vi "run control loops.vi"(6 "Reference Temperature [°F]":dbl, 8 "error in":errorcluster, 9 "Frequncy [Hz]":u16, 10 "input cluster":T1, 11 "dt [s]":dbl) -> (0 "error out":errorcluster, 1 "output cluster":T1, 2 "Duty Cycle Array":dbl[](array[numeric]), 3 "Temperature Array":dbl[](array[numeric]))   [LabVIEW 2025]
uses:
  Classes/controller/controller.lvclass
  Classes/hardware/hardware.lvclass
  Classes/data log/data log.lvclass
panel:
  in  "Hardware":refnum<class "hardware.lvclass">
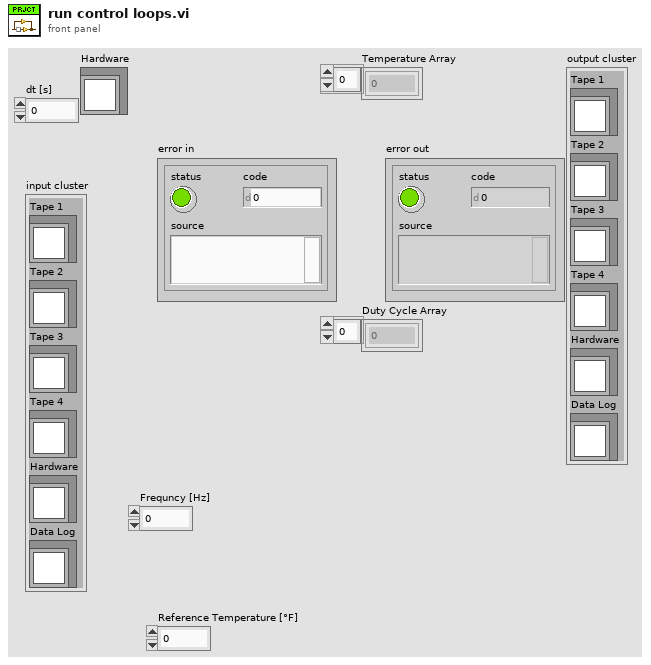
[diagram p1: front panel]
types:
  T1 = cluster{"Tape 1":refnum<class "controller.lvclass">, "Tape 2":refnum<class "controller.lvclass">, "Tape 3":refnum<class "controller.lvclass">, "Tape 4":refnum<class "controller.lvclass">, "Hardware":refnum<class "hardware.lvclass">, "Data Log":refnum<class "data log.lvclass">}
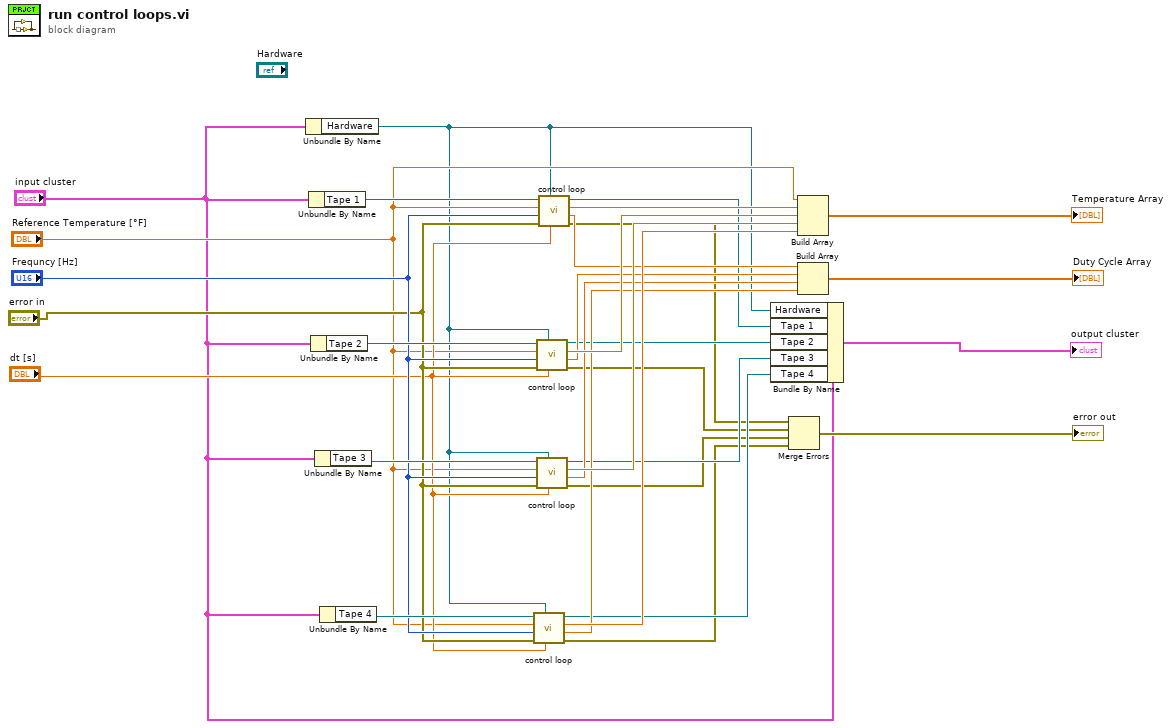
[diagram p0: block diagram]
diagram:
  n1 = Unbundle By Name("input cluster") -> ("Hardware"=w1:refnum<class "hardware.lvclass">)
  n2 = Unbundle By Name("input cluster") -> ("Tape 1"=w30:refnum<class "controller.lvclass">)
  n3 = Unbundle By Name("input cluster") -> ("Tape 2"=w29:refnum<class "controller.lvclass">)
  n4 = Unbundle By Name("input cluster") -> ("Tape 3"=w28:refnum<class "controller.lvclass">)
  n5 = Unbundle By Name("input cluster") -> ("Tape 4"=w27:refnum<class "controller.lvclass">)
  n6 = call-dynamic "control loop.vi"("dt [s]"="dt [s]", "Hardware"=w1, "error in (no error)"="error in", "Frequncey [Hz]"="Frequncy [Hz]", "Reference"="Reference Temperature [°F]", "controller in"=w27) -> ("error out"=w4:errorcluster, "input"=w14:dbl, "State"=w19:dbl, "controller out"=w9:refnum<class "controller.lvclass">)  [unwired: 2 in]
  n7 = call-dynamic "control loop.vi"("dt [s]"="dt [s]", "Hardware"=w1, "error in (no error)"="error in", "Frequncey [Hz]"="Frequncy [Hz]", "Reference"="Reference Temperature [°F]", "controller in"=w29) -> ("error out"=w6:errorcluster, "input"=w16:dbl, "State"=w21:dbl, "controller out"=w11:refnum<class "controller.lvclass">)  [unwired: 2 in]
  n8 = call-dynamic "control loop.vi"("dt [s]"="dt [s]", "Hardware"=w1, "error in (no error)"="error in", "Frequncey [Hz]"="Frequncy [Hz]", "Reference"="Reference Temperature [°F]", "controller in"=w28) -> ("error out"=w5:errorcluster, "input"=w15:dbl, "State"=w20:dbl, "controller out"=w10:refnum<class "controller.lvclass">)  [unwired: 2 in]
  n9 = call-dynamic "control loop.vi"("dt [s]"="dt [s]", "Hardware"=w1, "error in (no error)"="error in", "Frequncey [Hz]"="Frequncy [Hz]", "Reference"="Reference Temperature [°F]", "controller in"=w30) -> ("error out"=w7:errorcluster, "input"=w17:dbl, "State"=w22:dbl, "controller out"=w12:refnum<class "controller.lvclass">)  [unwired: 2 in]
  n10 = Bundle By Name(cluster="input cluster", "Hardware"=w1, "Tape 1"=w12, "Tape 2"=w11, "Tape 3"=w10, "Tape 4"=w9) -> (→"output cluster":T1)
  n11 = Merge Errors(w7, w6, w5, w4) -> (→"error out":errorcluster)
  n12 = Build Array("Reference Temperature [°F]", w22, w21, w20, w19) -> (→"Temperature Array":dbl[])
  n13 = Build Array(w17, w16, w15, w14) -> (→"Duty Cycle Array":dbl[])
